vi "libssh2_channel_process_startup.vi"(8 "error in (no error)":errorcluster, 9 "message":string, 10 "request":string, 11 "channel":T1) -> (0 "error out":errorcluster, 3 "return value":i32)   [LabVIEW 2013, in "libssh2.lvlib"]
doc: "Initiates a request on a session type channel."
uses:
  libssh2.lvlib
  Channel Refnum.ctl
  Global Settings.vi
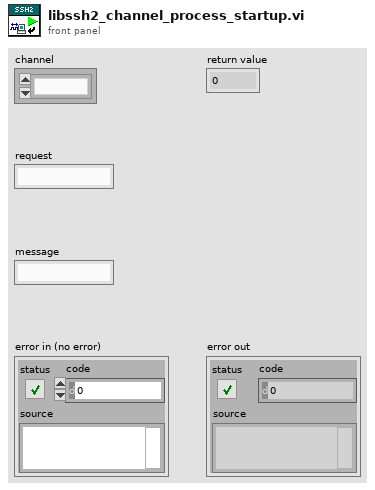
[diagram p1: front panel]
types:
  T1 = typedef "libssh2.lvlib/Channel Refnum.ctl" = refnum<k1>
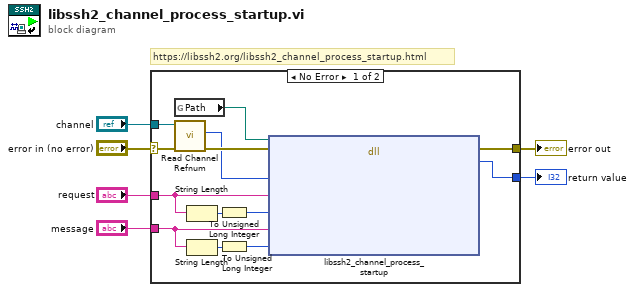
[diagram p0: block diagram]
diagram:
  # "https://libssh2.org/libssh2_channel_process_startup.html"
  n1 = case shown="No Error" "error in (no error)" {
    selector: "error in (no error)" -> [w8 w20]
    tunnel: "request" -> [w19 _]
    tunnel: "message" -> [w16 _]
    tunnel: [w15 _] -> w4
    tunnel: [w14 w20] -> w3
    tunnel: "channel" -> [w11 _]
    frame No Error {
      n2 = global read "Global Settings.vi" "Path"() -> (w7:path)
      n3 = call "Read Channel Refnum.vi"("error in (no error)"=w8, "channel"=w11) -> ("error out"=w13:errorcluster, "LIBSSH2_CHANNEL*"=w12:u64)  [unwired: 8 in]
      n4 = String Length(string=w19) -> (length=w10:i32)
      n5 = String Length(string=w16) -> (length=w9:i32)
      n6 = To Unsigned Long Integer(number=w10) -> (unsigned 32bit integer=w18:u32)
      n7 = To Unsigned Long Integer(number=w9) -> (unsigned 32bit integer=w17:u32)
      n8 = dll-call lib="C:/Users/pasca/source/repos/libssh2-labview/libssh2/libssh2**.*" fn="libssh2_channel_process_startup"(path in=w7, error in=w13, "channel"=w12, "request"=w19, "request_len"=w18, "message"=w16, "message_len"=w17) -> (error out=w14:errorcluster, "return value"=w15:i32)  [unwired: 6 in, 1 out]
    }
    frame Error {
    }
  }
  "return value" <- w4
  "error out" <- w3
